vi "saveImages.vi"(7 "totalImageNumber":i32, 8 "error in (no error)":errorcluster, 9 "U16bit image data":u16[][](array[numeric]), 10 "Path":path, 11 "ProEM_WinX32 in":refnum<class "ProEM_WinX32.lvclass">) -> (0 "error out":errorcluster, 3 "ProEM_WinX32 out":refnum<class "ProEM_WinX32.lvclass">)   [LabVIEW 2009, in "Hardware.lvlib" / "Channels.lvlib" / "ProEM_WinX32.lvclass"]
uses:
  ProEM_WinX32.lvclass
  Camera/Camera.lvclass
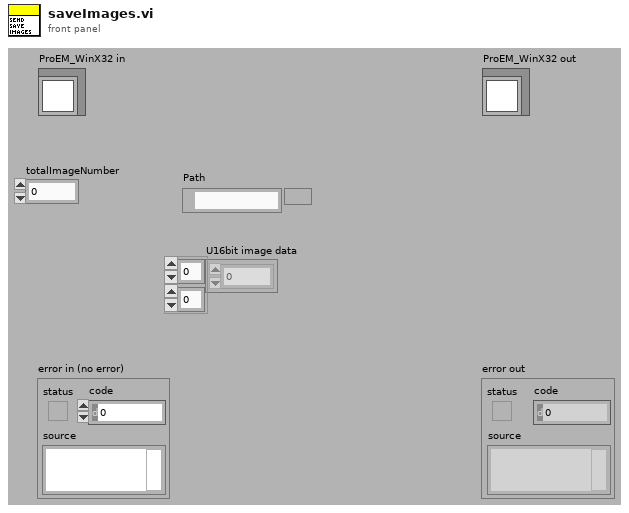
[diagram p1: front panel]
types:
  T1 = cluster{"cameraType":string, "imageName":string, "saved":string, "analysisType":string, "U16bit image data":u16[][], "path":path}
  T2 = typedef "Image Type" = u32
  T3 = typedef "IMAQ Image.ctl" = refnum<image>
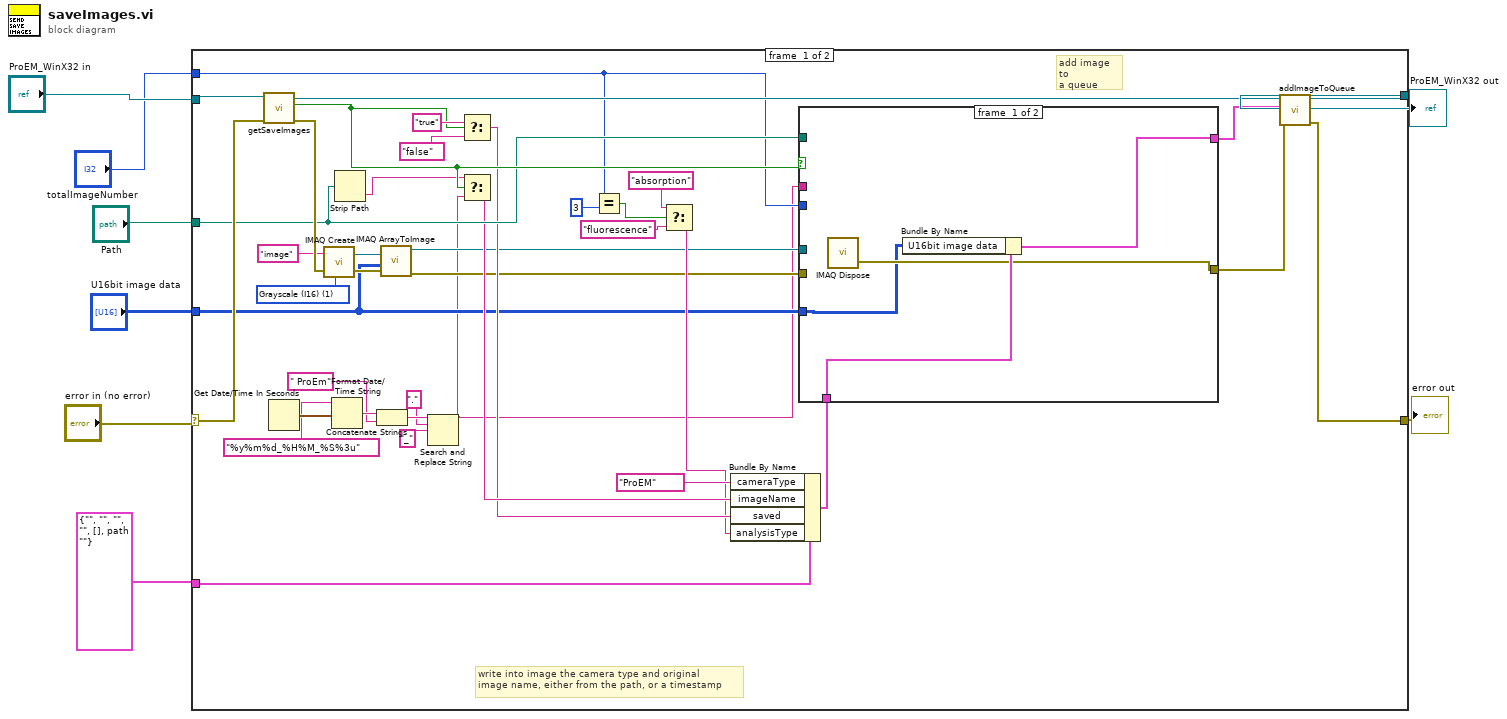
[diagram p0: block diagram]
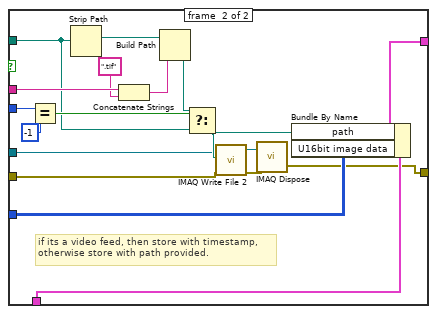
[diagram p2: hidden frame]
diagram:
  n1 = case shown="No Error" "error in (no error)" {
    selector: "error in (no error)" -> [w47 w71]
    tunnel: [w39 w71] -> w6
    tunnel: [w40 w70] -> w5
    tunnel: "ProEM_WinX32 in" -> [w31 w70]
    tunnel: "Path" -> [w25 _]
    tunnel: "U16bit image data" -> [w15 _]
    tunnel: "totalImageNumber" -> [w23 _]
    tunnel: T1 {"cameraType"="", "imageName"="", "saved"="", "analysisType"="", "U16bit image data"=[], "path"=path ""} ("ImageData") -> [w22 _]
    frame #0 {
      w44 = T2 1 items=["Grayscale (U8)", "Grayscale (I16)", "Grayscale (SGL)", "Complex (CSG)", "RGB (U32)", "HSL (U32)", "RGB (U64)", "Grayscale (U16)"] ("Image Type")
      # "write into image the camera type and original\nimage name, either from the path, or a timestamp"
      # "add image to\na queue"
      n2 = call "getSaveImages.vi"("error in (no error)"=w47, "Camera in"=w31) -> ("error out"=w46:errorcluster, "saveImages?"=w26:bool, "Camera out"=w41:refnum<class "ProEM_WinX32.lvclass">)  [unwired: 7 in]
      n3 = Get Date/Time In Seconds() -> (seconds since 1Jan1904=w38:timestamp)
      n4 = call "IMAQ Create"("Image Name"="image", "Image Type"=w44, "error in (no error)"=w46) -> ("New Image"=w43:T3, "error out"=w42:errorcluster)  [unwired: 2 in]
      n5 = Format Date/Time String(time format string (%c)="%y%m%d_%H%M_%S%3u", seconds (now)=w38) -> (date/time string=w36:string)  [unwired: 1 in]
      n6 = Strip Path(path=w25) -> (name=w24:string)  [unwired: 1 out]
      n7 = Concatenate Strings(w36, " ProEm") -> (w12:string)
      n8 = call "IMAQ ArrayToImage"("error in (no error)"=w42, "Image Pixels (I16)"=w15, "Image"=w43) -> ("error out"=w13:errorcluster, "Image Out"=w14:T3)  [unwired: 7 in]
      n9 = Search and Replace String(input string=w12, search string=".", replace string="_") -> (result string=w11:string)  [unwired: 5 in, 3 out]
      n10 = Select(t="true", s=w26, f="false") -> (s? t:f=w19:string)
      n11 = Select(t=w24, s=w26, f=w11) -> (s? t:f=w20:string)
      n12 = Equal?(x=w23, y=3) -> (x = y?=w29:bool)
      n13 = Select(t="absorption", s=w29, f="fluorescence") -> (s? t:f=w18:string)
      n14 = Bundle By Name(cluster=w22, "cameraType"="ProEM", "imageName"=w20, "saved"=w19, "analysisType"=w18) -> (w17:T1)
      n15 = case shown="True" w26 {
        tunnel: [w49 w54] -> w32
        tunnel: [w50 w59] -> w16
        tunnel: w25 -> [_ w62]
        tunnel: w11 -> [_ w68]
        tunnel: w23 -> [_ w61]
        tunnel: w17 -> [w51 w60]
        tunnel: w15 -> [w48 w57]
        tunnel: w14 -> [_ w53]
        tunnel: w13 -> [_ w52]
        frame #0 {
          n16 = call "IMAQ Dispose"() -> ("error out"=w49:errorcluster)  [unwired: 6 in]
          n17 = Bundle By Name(cluster=w51, "U16bit image data"=w48) -> (w50:T1)
        }
        frame #1 {
          # "if its a video feed, then store with timestamp,\notherwise store with path provided."
          n18 = Equal?(x=w61, y=-1) -> (x = y?=w63:bool)
          n19 = Strip Path(path=w62) -> (stripped path=w69:path)  [unwired: 1 out]
          n20 = Concatenate Strings(w68, ".tif") -> (w66:string)
          n21 = Build Path(base path=w69, name or relative path=w66) -> (appended path=w64:path)
          n22 = Select(t=w64, s=w63, f=w62) -> (s? t:f=w58:path)
          n23 = call-poly "IMAQ Write File 2"("error in (no error)"=w52, "File Path"=w58, "Image"=w53) -> ("error out"=w56:errorcluster, "Image Out (duplicate)"=w55:T3)  [unwired: 7 in]
          n24 = call "IMAQ Dispose"("Image"=w55, "error in (no error)"=w56) -> ("error out"=w54:errorcluster)  [unwired: 4 in]
          n25 = Bundle By Name(cluster=w60, "path"=w58, "U16bit image data"=w57) -> (w59:T1)
        }
      }
      n26 = call "addImageToQueue.vi"("error in (no error)"=w32, "ImageData"=w16, "Camera in"=w41) -> ("error out"=w39:errorcluster, "Camera out"=w40:refnum<class "ProEM_WinX32.lvclass">)  [unwired: 7 in]
    }
    frame #1 {
    }
  }
  "error out" <- w6
  "ProEM_WinX32 out" <- w5
